vi "Old_main_broken.vi"() -> ()   [LabVIEW 2019]
uses:
  Control 3.ctl
  Control 1.ctl
  <vilib>/Analysis/3filter.llb/Filter Passband Type.ctl
  <vilib>/Analysis/5stat.llb/RMS (DBL).vi
  <vilib>/Analysis/3filter.llb/Butterworth Filter (DBL).vi
  <vilib>/Analysis/NI_AALPro.lvlib
  <vilib>/Analysis/NI_AALBase.lvlib
panel:
  out "Prubehy RMS":cluster{"rms value":dbl, "rms value":dbl}(graph)
  in  "Citlivost vypoctu frekvence":i32=10
  in  "Citlivost vypoctu frekvence":i32=50
  out "Perioda ze spektra.":dbl
  out "Perioda ze spektra":dbl
  out "Ursm":dbl format="%0.2f"
  out "Perioda z pruchodu nulou":dbl
  out "Frekvence z pruchodu nulou":dbl
  out "Urms":dbl format="%0.2f"
  out "Perioda z pruchodu nulou.":dbl
  out "Frekvence z pruchodu nulou.":dbl
  out "Frekvence ze spektra":i32
  out "Frekvence ze spektra.":i32
  out "Spektrum puvodniho signalu":cluster{dbl[], dbl[]}(graph)
  out "Spektrum prevzorkovaneho signalu":cluster{dbl[], dbl[]}(graph)
  out "Prevzorkovany signal":waveform(dbl)(graph)
  in  "Napetovy treshold":dbl=10.0
  in  "Úroven filtrace":i32
  out "Triggered signal":cluster{dbl[], "Vstupní pole":dbl[]}(graph)
  out "SamInWin":i32
  in  "Sirka okna (ms)":i32(listbox)=1
  in  "Offset":dbl format="%0.2p"
  in  "Amplituda sumu":T1
  in  "Amplituda":dbl=1.0 format="%0.2p"
  in  "Frekvence":dbl=10.0 format="%0.2p"
  out "Signal z generatoru":waveform(dbl)(graph)
  out "dt":dbl
  in  "stop":bool
  # "Parametry generatoru signalu"
  # "Hide!"
  # "Parametry navzorkovaneho signalu"
  # "Parametry prevzorkovaneho signalu"
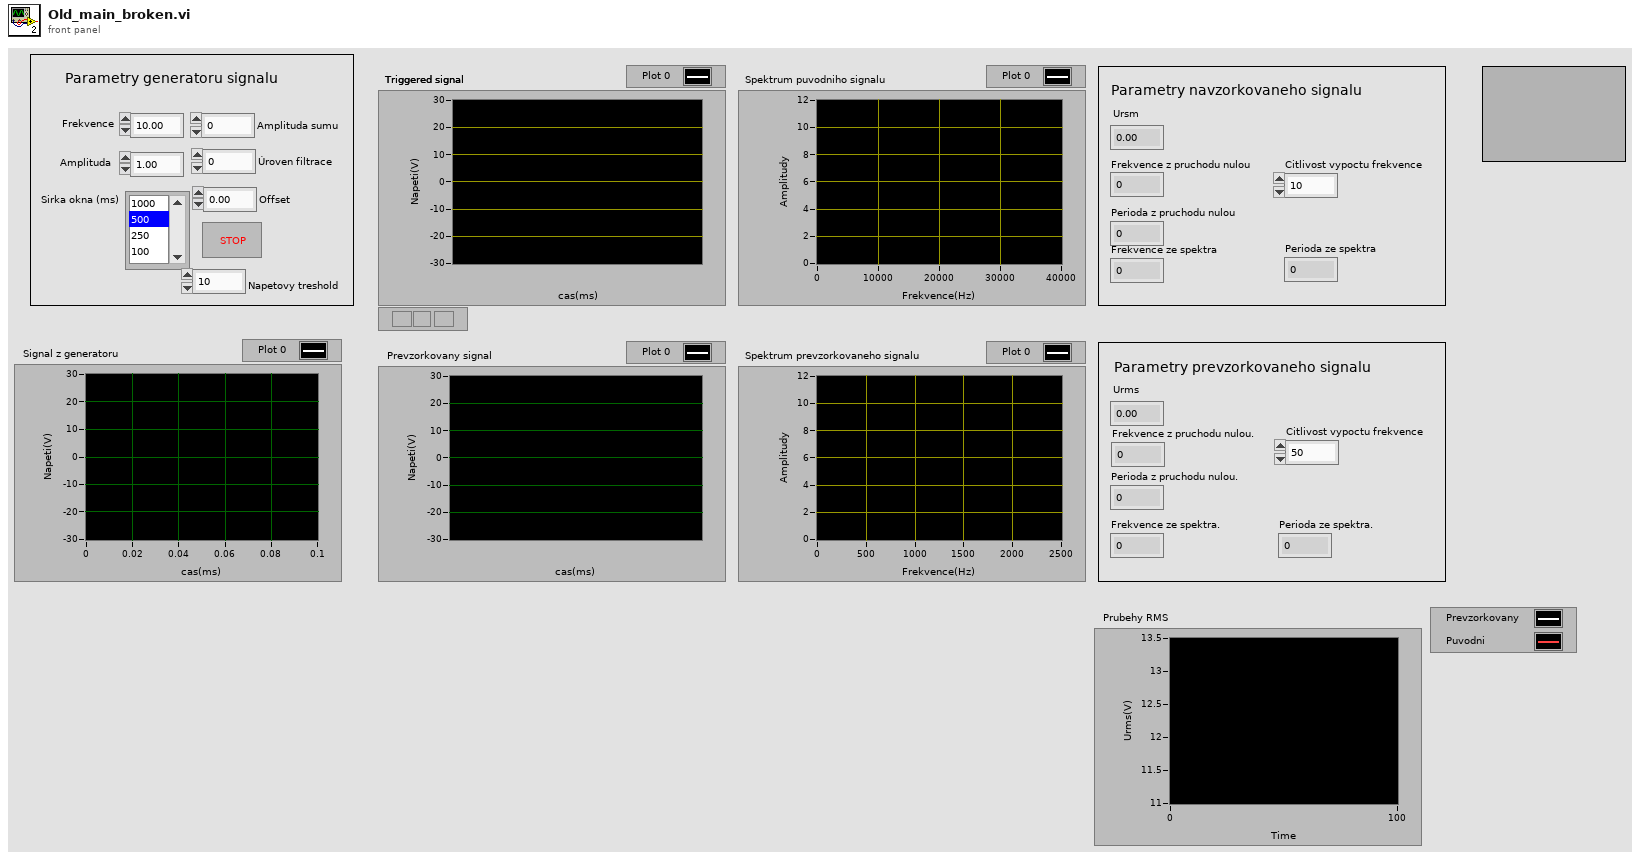
[diagram p1: front panel]
types:
  T1 = typedef "Control 3.ctl" = dbl
  T2 = enum16{"open", "open or create", "create or replace", "create", "open (read-only)"}
  T3 = cluster{"Waveform":waveform(dbl), "Waveform":waveform(dbl), "Waveform":waveform(dbl), "seconds since 1Jan1904":timestamp, bool, bool}
  T4 = typedef "Control 1.ctl" = dbl
  T5 = cluster{"name (unnamed)":string, "Variant":variant}
  T6 = typedef "NI_AALBase.lvlib/Filter Passband Type.ctl" = enum32{"Lowpass", "Highpass", "Bandpass", "Bandstop"}
  T7 = cluster{waveform(dbl), waveform(dbl), waveform(dbl), "seconds since 1Jan1904":timestamp, bool, bool}
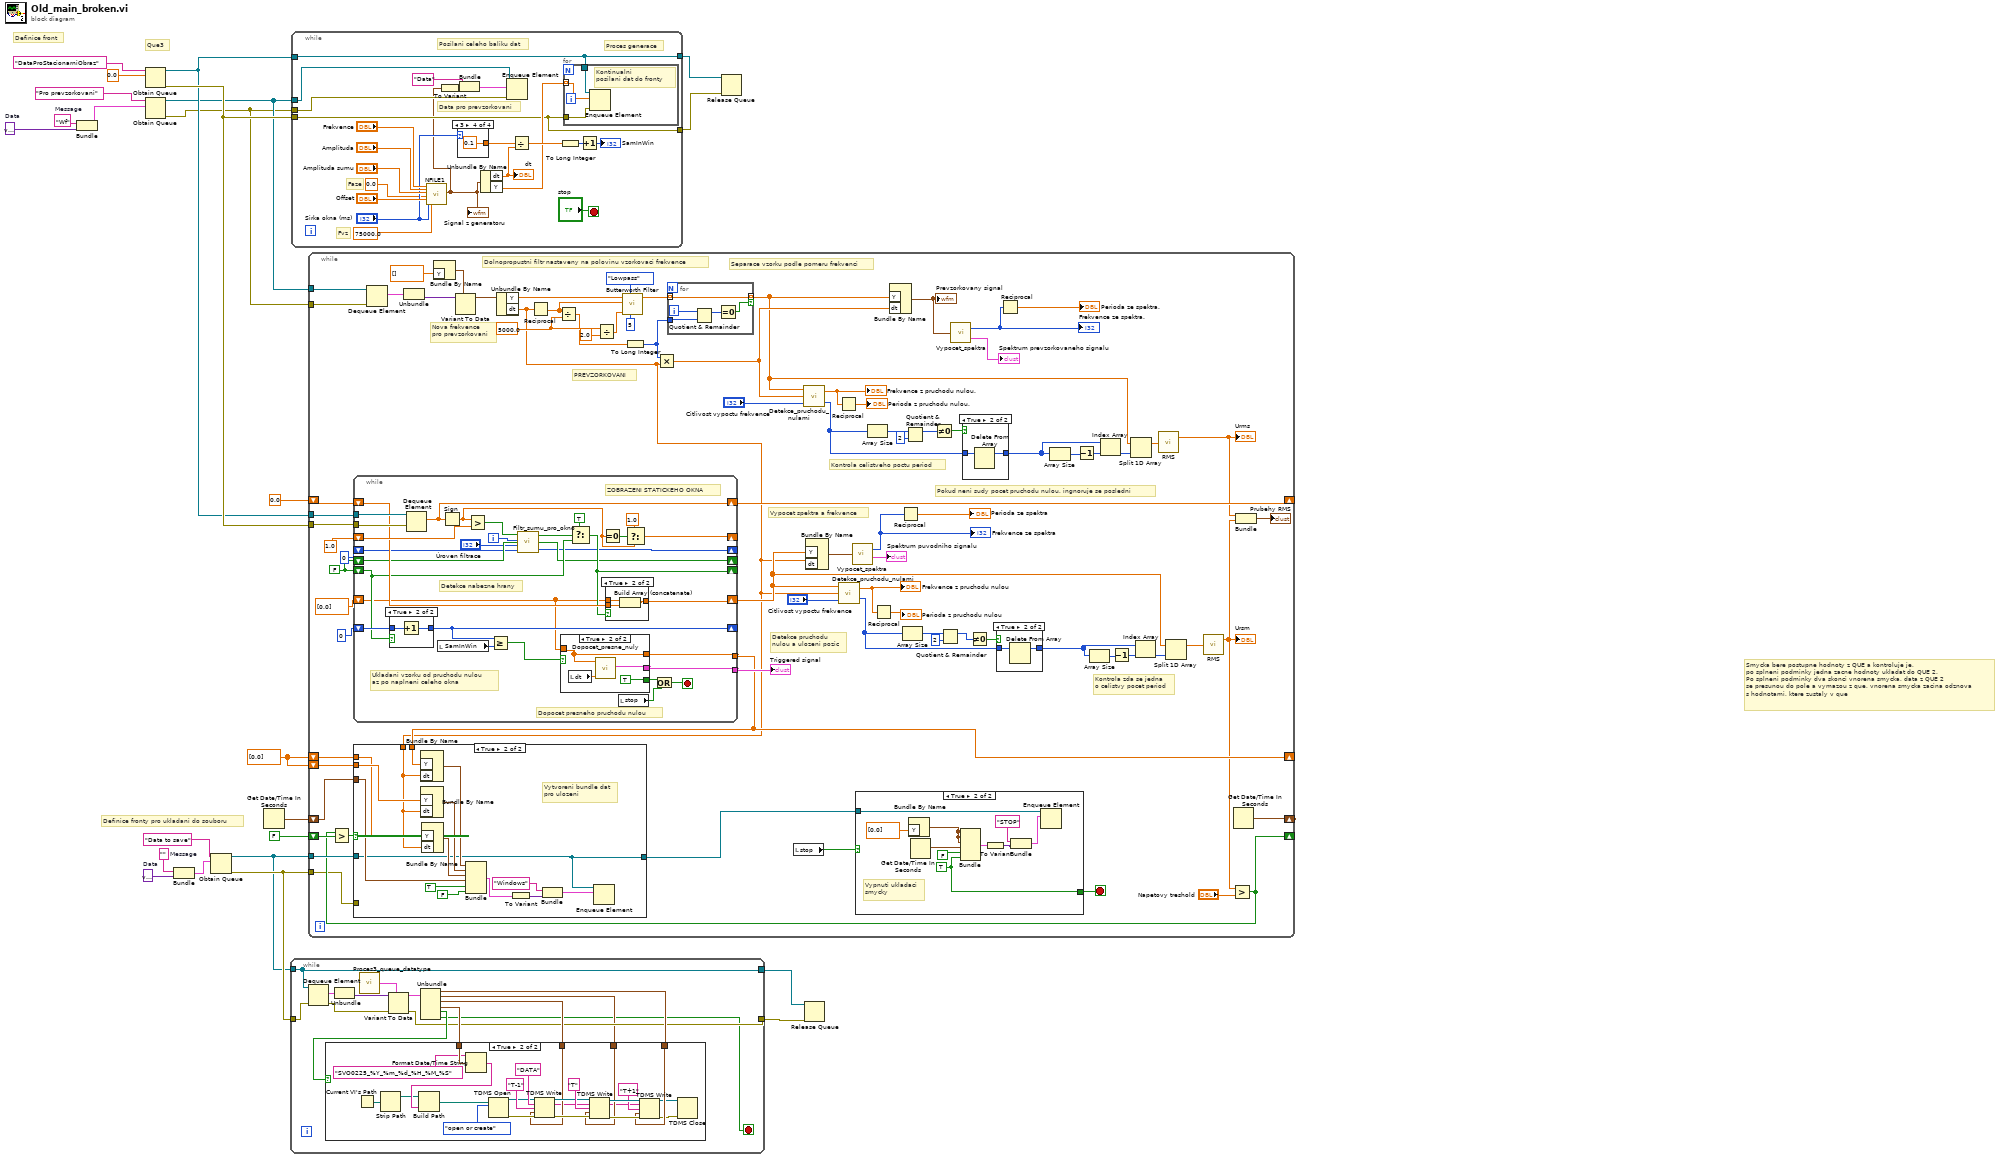
[diagram p0: block diagram]
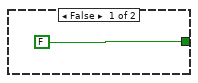
[diagram p3: hidden frame]
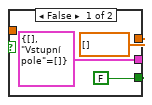
[diagram p6: hidden frame]
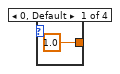
[diagram p10: hidden frame]
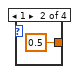
[diagram p11: hidden frame]
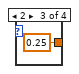
[diagram p12: hidden frame]
diagram:
  w2 = dbl[] [0.0]
  w1 = variant  # Data
  w6 = "Wf"  # Message
  w17 = variant  # Data
  w18 = ""  # Message
  # "Definice fronty pro ukladani do souboru"
  # "Definice front"
  # "Que3"
  # "Smycka bere postupne hodnoty z QUE a kontroluje je,\npo splneni podminky jedna zacne hodnoty ukladat do QUE 2.\nPo splneni podminky dva skonci vnorena smycka, data z QUE 2 \nse presunou do pole a vymazou z que, vnorena smycka zacina odznova\ns hodnotami, ktere zustaly v que"
  n1 = Bundle("Message"=w6, "Data"=w1) -> (w5:cluster{"Message":string, "Data":variant})  [unwired: 1 in]
  n2 = Obtain Queue(name (unnamed)="DataProStacionarniObraz", element data type=0.0) -> (queue out=w21:refnum<queue>, error out=w22:errorcluster)  [unwired: 3 in, 1 out]
  n3 = Obtain Queue(name (unnamed)="Pro prevzorkovani", element data type=w5) -> (queue out=w8:refnum<queue>, error out=w7:errorcluster)  [unwired: 3 in, 1 out]
  n4 = Bundle("Message"=w18, "Data"=w17) -> (w16:cluster{"Message":string, "Data":variant})  [unwired: 1 in]
  n5 = Obtain Queue(name (unnamed)="Data to save", element data type=w16) -> (queue out=w13:refnum<queue>, error out=w14:errorcluster)  [unwired: 3 in, 1 out]
  n6 = Get Date/Time In Seconds() -> (seconds since 1Jan1904=w3:timestamp)
  n7 = while {
    tunnel: w14 -> [w29]
    tunnel: w13 -> [w34]
    tunnel: [w34] -> w12
    tunnel: [w27] -> w11
    stop <- w25 stop-if-true
    n8 = Dequeue Element(queue=w34, error in (no error)=w29) -> (element=w38:cluster{"Message":string, "Data":variant}, error out=w28:errorcluster)  [unwired: 1 in, 2 out]
    n9 = Unbundle(w38) -> ("Data"=w37:variant)  [unwired: 1 out]
    n10 = call "Proces3_queue_datatype.vi"() -> ("output cluster"=w36:T3)  [unwired: 1 in]
    n11 = Variant To Data(error in=w28, type=w36, Variant=w37) -> (data=w35:T3, error out=w27:errorcluster)
    n12 = Unbundle(w35) -> ("Waveform"=w33:waveform(dbl), "Waveform"=w26:waveform(dbl), "Waveform"=w30:waveform(dbl), "seconds since 1Jan1904"=w32:timestamp, w31:bool, w25:bool)
    n13 = case shown="True" w31 {
      tunnel: w33 -> [_ w51]
      tunnel: w32 -> [_ w50]
      tunnel: w30 -> [_ w44]
      tunnel: w26 -> [_ w43]
      frame False {
      }
      frame True {
        n14 = Current VI's Path() -> (path=w62:path)
        n15 = Strip Path(path=w62) -> (stripped path=w39:path)  [unwired: 1 out]
        n16 = Format Date/Time String(time format string (%c)="SVO0225_%Y_%m_%d_%H_%M_%S", seconds (now)=w50) -> (date/time string=w61:string)  [unwired: 1 in]
        n17 = Build Path(base path=w39, name or relative path=w61) -> (appended path=w60:path)
        n18 = TDMS Open(10:T2."open or create" ("operation (0:open)"), 11:w60) -> (0:w55:errorcluster, 3:w56:refnum<k34>)  [unwired: 5 in]
        n19 = TDMS Write(0:w56, 5:"DATA" ("group name in (Untitled)"), 7:"T-1", 9:w44, 11:w55) -> (4:w45:refnum<k34>, 6:w42:string, 15:w54:errorcluster)  [unwired: 1 in, 1 out]
        n20 = TDMS Write(0:w45, 5:w42, 7:"T", 9:w43, 11:w54) -> (4:w46:refnum<k34>, 6:w40:string, 15:w52:errorcluster)  [unwired: 1 in, 1 out]
        n21 = TDMS Write(0:w46, 5:w40, 7:"T+1", 9:w51, 11:w52) -> (4:w48:refnum<k34>, 15:w49:errorcluster)  [unwired: 1 in, 2 out]
        n22 = TDMS Close(8:w49, 11:w48) -> ()  [unwired: 2 out]
      }
    }
  }
  n23 = while {
    tunnel: w22 -> [w70]
    tunnel: w21 -> [w71]
    tunnel: [w71] -> w10
    tunnel: [w70] -> w9
    tunnel: w8 -> [w69]
    tunnel: w7 -> [w68]
    stop <- "stop" stop-if-true
    # "Posilani celeho baliku dat"
    # "Data pro prevzorkovani"
    # "Proces generace"
    # "Fvz"
    # "Faze"
    n24 = call "NFILE1.vi"("Frekvence"="Frekvence", "Amplituda"="Amplituda", "Amplituda sumu"="Amplituda sumu", "Fáze"=0.0, "Offset"="Offset", "Sirka okna (ms)"="Sirka okna (ms)", "Fvz"=T4 75000.0) -> ("Waveform Graph"=w65:waveform(dbl))  [unwired: 12 in]
    "Signal z generatoru" <- w65
    n25 = To Variant(anything=w65) -> (Variant=w66:variant)
    n26 = case shown="3" "Sirka okna (ms)" {
      tunnel: [1.0 ("X Scale.Range:Maximum") 0.5 ("X Scale.Range:Maximum") 0.25 ("X Scale.Range:Maximum") 0.1 ("X Scale.Range:Maximum")] -> w77
      frame 0, Default {
      }
      frame 1 {
      }
      frame 2 {
      }
      frame 3 {
      }
    }
    n27 = Bundle("name (unnamed)"="Data", "Variant"=w66) -> (w67:T5)  [unwired: 1 in]
    n28 = Unbundle By Name(w65) -> ("dt"=w63:dbl, "Y"=w74:dbl[])
    "dt" <- w63
    n29 = Enqueue Element(queue=w69, element=w67, error in (no error)=w68) -> ()  [unwired: 1 in, 3 out]
    n30 = Divide(x=w77, y=w63) -> (x/y=w76:dbl)
    n31 = To Long Integer(number=w76) -> (32bit integer=w73:i32)
    n32 = for {
      tunnel: w70 -> [w87]
      tunnel: w71 -> [w86]
      tunnel: w74 -> [w85] mode=indexing
      # "Kontinualni\nposilani dat do fronty"
      n33 = Enqueue Element(queue=w86, element=w85, error in (no error)=w87) -> ()  [unwired: 1 in, 3 out]
    }
    n34 = Increment(x=w73) -> (x+1=→"SamInWin":i32)
  }
  n35 = while {
    tunnel: w22 -> [w173]
    tunnel: w21 -> [w172]
    shift-right: [w169] -> _
    shift-left: 0.0 -> [w168]
    shift-right: [w109] -> _
    shift-left: w2 -> [w164]
    shift-left: w2 -> [w163]
    shift-right: [w123] -> _
    shift-left: FALSE -> [w161]
    tunnel: w13 -> [w165]
    tunnel: w14 -> [w95]
    tunnel: w8 -> [w160]
    tunnel: w7 -> [w159]
    shift-right: [w100] -> _
    shift-left: w3 -> [w99]
    stop <- w94 stop-if-true
    w150 = T4 5000.0 ("Fvz")
    w97 = FALSE
    # "PREVZORKOVANI"
    # "Vypocet spektra a frekvence"
    # "Detekce pruchodu\nnulou a ulozeni pozic"
    # "Pokud neni sudy pocet pruchodu nulou, ingnoruje se posledni"
    # "Kontrola celistveho poctu period"
    # "Separace vzorku podle pomeru frekvenci"
    # "Dolnopropustni filtr nastaveny na polovinu vzorkovaci frekvence"
    # "Nova frekvence\npro prevzorkovani"
    # "Kontrola zda se jedna\no celistvy pocet period"
    n36 = while {
      tunnel: w172 -> [w234]
      tunnel: w173 -> [w233]
      shift-right: [w215] -> _
      shift-left: 1.0 -> [w232]
      shift-right: [w228] -> _
      shift-left: 0 -> [w230]
      shift-right: [w214] -> w108
      shift-left: dbl[] [0.0] -> [w211]
      tunnel: [w227] -> w170
      shift-right: [w224] -> _
      shift-left: w97 -> [w225]
      shift-right: [w213] -> w169
      shift-left: w168 -> [w226]
      shift-right: [w220] -> _
      shift-left: w97 -> [w221]
      tunnel: [w212] -> w109
      shift-right: [w209] -> _
      shift-left: 0 -> [w210]
      i -> [w222]
      stop <- w207 stop-if-true
      # "ZOBRAZENI STATICKEHO OKNA"
      # "Dopocet presneho pruchodu nulou"
      # "Detekce nabezne hrany"
      # "Ukladani vzorku od pruchodu nulou\naz po naplneni celeho okna"
      n37 = case shown="True" w225 {
        tunnel: w230 -> [w242 w244]
        tunnel: [w242 w243] -> w228
        frame False {
        }
        frame True {
          n38 = Increment(x=w244) -> (x+1=w243:i32)
        }
      }
      n39 = Dequeue Element(queue=w234, error in (no error)=w233) -> (element=w213:dbl)  [unwired: 1 in, 3 out]
      n40 = local read "SamInWin"() -> (w229:i32)
      n41 = Sign(1:w213) -> (0:w204:dbl)
      n42 = Greater?(x=w204, y=w232) -> (0:w223:bool)
      n43 = Greater Or Equal?(x=w228, y=w229) -> (x >= y?=w218:bool)
      n44 = call "Filtr_sumu_pro_okno.vi"("trig_in"=w223, "i"=w222, "Citlivost 2"="Úroven filtrace", "BShitftIn"=w210, "ShiftIn"=w221) -> ("trig_out"=w219:bool, "ShiftOut"=w220:bool, "BShiftOut"=w209:i32)
      n45 = case shown="True" w218 {
        tunnel: [FALSE TRUE] -> w206
        tunnel: w211 -> [_ w238]
        tunnel: [cluster{dbl[], "Vstupní pole":dbl[]} {[], "Vstupní pole"=[]} ("XY Graph 2") w239] -> w227
        tunnel: [dbl[] [] w238] -> w212
        frame False {
        }
        frame True {
          n46 = local read "dt"() -> (w240:dbl)
          n47 = call "Dopocet_presne_nuly.vi"("dt"=w240, "Vstupní pole"=w238) -> ("XY Graph"=w239:cluster{dbl[], "Vstupní pole":dbl[]})  [unwired: 9 in]
        }
      }
      n48 = Select(t=TRUE, s=w219, f=w225) -> (s? t:f=w224:bool)
      n49 = Equal To 0?(x=w204) -> (x = 0?=w217:bool)
      n50 = case shown="True" w224 {
        tunnel: w211 -> [w245 w248]
        tunnel: w226 -> [_ w247]
        tunnel: [w245 w246] -> w214
        frame False {
        }
        frame True {
          n51 = Build Array (concatenate)(w248, w247) -> (w246:dbl[])
        }
      }
      n52 = local read "stop"() -> (w205:bool)
      n53 = Select(t=1.0, s=w217, f=w204) -> (s? t:f=w215:dbl)
      n54 = Or(x=w206, y=w205) -> (x .or. y?=w207:bool)
    }
    "Triggered signal" <- w170
    n55 = Dequeue Element(queue=w160, error in (no error)=w159) -> (element=w158:cluster{"Message":string, "Data":variant})  [unwired: 1 in, 3 out]
    n56 = Unbundle(w158) -> ("Data"=w157:variant)  [unwired: 1 out]
    n57 = Bundle By Name("Y"=dbl[] []) -> (w156:waveform(dbl))  [unwired: 1 in]
    n58 = Variant To Data(type=w156, Variant=w157) -> (data=w155:waveform(dbl))  [unwired: 1 in, 1 out]
    n59 = Unbundle By Name(w155) -> ("Y"=w144:dbl[], "dt"=w98:dbl)
    n60 = Reciprocal(x=w98) -> (1/x=w149:dbl)
    n61 = Divide(x=w149, y=w150) -> (x/y=w147:T4)
    n62 = Divide(x=w150, y=2.0) -> (x/y=w153:T4)
    n63 = call-poly <vilib>:"Butterworth Filter.vi"("order"=5, "filter type"=Filter_Passband_Type."Lowpass", "low cutoff freq: fl"=w153, "sampling freq: fs"=w149, "X"=w144) -> ("Filtered X"=w148:dbl[])  [unwired: 3 in, 1 out]
    n64 = To Long Integer(number=w147) -> (32bit integer=w146:i32)
    n65 = Multiply(x=w146, y=w98) -> (x*y=w138:dbl)
    n66 = for {
      tunnel: w148 -> [w253] mode=indexing
      tunnel: w146 -> [w255]
      tunnel: [w253] -> w125 mode=indexing if=w252
      i -> [w256]
      n67 = Quotient & Remainder(x=w256, y=w255) -> (x-y*floor(x/y)=w254:i32)  [unwired: 1 out]
      n68 = Equal To 0?(x=w254) -> (x = 0?=w252:bool)
    }
    n69 = local read "stop"() -> (w93:bool)
    n70 = call "Detekce_pruchodu_nulami.vi"("Citlivost vypoctu frekvence"="Citlivost vypoctu frekvence", "dt 2"=w138, "array"=w125) -> ("Pole indexu pruchodu nulou"=w130:i32[], "Numeric"=w135:dbl)
    "Frekvence z pruchodu nulou." <- w135
    n71 = Bundle By Name("Y"=w108, "dt"=w98) -> (w142:waveform(dbl))  [unwired: 1 in]
    n72 = Reciprocal(x=w135) -> (1/x=→"Perioda z pruchodu nulou.":dbl)
    n73 = call "Detekce_pruchodu_nulami.vi"("Citlivost vypoctu frekvence"="Citlivost vypoctu frekvence", "dt 2"=w98, "array"=w108) -> ("Pole indexu pruchodu nulou"=w115:i32[], "Numeric"=w120:dbl)
    "Frekvence z pruchodu nulou" <- w120
    n74 = call "Vypocet_spektra.vi"("waveform"=w142) -> ("Frekvence"=w107:i32, "XY Graph"=→"Spektrum puvodniho signalu":cluster{dbl[], dbl[]})
    "Frekvence ze spektra" <- w107
    n75 = Array Size(array=w130) -> (size(s)=w133:i32)
    n76 = Reciprocal(x=w120) -> (1/x=→"Perioda z pruchodu nulou":dbl)
    n77 = Bundle By Name("Y"=w125, "dt"=w138) -> (w143:waveform(dbl))  [unwired: 1 in]
    "Prevzorkovany signal" <- w143
    n78 = Reciprocal(x=w107) -> (1/x=→"Perioda ze spektra":dbl)
    n79 = Array Size(array=w115) -> (size(s)=w118:i32)
    n80 = Quotient & Remainder(x=w133, y=2) -> (x-y*floor(x/y)=w134:i32)  [unwired: 1 out]
    n81 = Not Equal To 0?(x=w134) -> (x != 0?=w131:bool)
    n82 = Quotient & Remainder(x=w118, y=2) -> (x-y*floor(x/y)=w119:i32)  [unwired: 1 out]
    n83 = call "Vypocet_spektra.vi"("waveform"=w143) -> ("Frekvence"=w104:i32, "XY Graph"=→"Spektrum prevzorkovaneho signalu":cluster{dbl[], dbl[]})
    "Frekvence ze spektra." <- w104
    n84 = case shown="True" w131 {
      tunnel: w130 -> [w249 w251]
      tunnel: [w249 w250] -> w127
      frame False {
      }
      frame True {
        n85 = Delete From Array(array=w251) -> (array with subset deleted=w250:i32[])  [unwired: 2 in, 1 out]
      }
    }
    n86 = Not Equal To 0?(x=w119) -> (x != 0?=w116:bool)
    n87 = case shown="True" w116 {
      tunnel: w115 -> [w185 w187]
      tunnel: [w185 w186] -> w112
      frame False {
      }
      frame True {
        n88 = Delete From Array(array=w187) -> (array with subset deleted=w186:i32[])  [unwired: 2 in, 1 out]
      }
    }
    n89 = Reciprocal(x=w104) -> (1/x=→"Perioda ze spektra.":dbl)
    n90 = Array Size(array=w127) -> (size(s)=w129:i32)
    n91 = Decrement(x=w129) -> (x-1=w128:i32)
    n92 = Array Size(array=w112) -> (size(s)=w114:i32)
    n93 = Index Array(array=w127, index=w128) -> (element=w126:i32)
    n94 = Decrement(x=w114) -> (x-1=w113:i32)
    n95 = Split 1D Array(array=w125, index=w126) -> (first subarray=w124:dbl[])  [unwired: 1 out]
    n96 = Index Array(array=w112, index=w113) -> (element=w111:i32)
    n97 = call-poly <vilib>:"RMS.vi"("X"=w124) -> ("rms value"=w102:dbl)  [unwired: 1 out]
    "Urms" <- w102
    n98 = Split 1D Array(array=w108, index=w111) -> (first subarray=w110:dbl[])  [unwired: 1 out]
    n99 = call-poly <vilib>:"RMS.vi"("X"=w110) -> ("rms value"=w103:dbl)  [unwired: 1 out]
    "Ursm" <- w103
    n100 = Greater?(x=w103, y="Napetovy treshold") -> (0:w123:bool)
    n101 = Greater?(x=w123, y=w161) -> (0:w162:bool)
    n102 = case shown="True" w162 {
      tunnel: w165 -> [w188 w189]
      tunnel: w164 -> [_ w196]
      tunnel: w163 -> [_ w197]
      tunnel: w109 -> [_ w198]
      tunnel: w99 -> [_ w199]
      tunnel: w98 -> [_ w195]
      tunnel: w95 -> [_ _]
      tunnel: [w188 w189] -> w92
      frame False {
      }
      frame True {
        # "Vytvoreni bundle dat\npro ulozeni"
        n103 = Bundle By Name("Y"=w198, "dt"=w195) -> (w192:waveform(dbl))  [unwired: 1 in]
        n104 = Bundle By Name("Y"=w197, "dt"=w195) -> (w193:waveform(dbl))  [unwired: 1 in]
        n105 = Bundle By Name("Y"=w196, "dt"=w195) -> (w194:waveform(dbl))  [unwired: 1 in]
        n106 = Bundle(w192, w193, w194, "seconds since 1Jan1904"=w199, TRUE, FALSE) -> (w201:T7)  [unwired: 1 in]
        n107 = To Variant(anything=w201) -> (Variant=w202:variant)
        n108 = Bundle("Windows", "Variant"=w202) -> (w200:cluster{string, "Variant":variant})  [unwired: 1 in]
        n109 = Enqueue Element(queue=w189, element=w200) -> ()  [unwired: 2 in, 3 out]
      }
    }
    n110 = case shown="True" w93 {
      tunnel: [FALSE w181] -> w94
      tunnel: w92 -> [_ w179]
      frame False {
      }
      frame True {
        w181 = TRUE
        # "Vypnuti ukladaci\nsmycky"
        n111 = Bundle By Name("Y"=dbl[] [0.0]) -> (w184:waveform(dbl))  [unwired: 1 in]
        n112 = Get Date/Time In Seconds() -> (seconds since 1Jan1904=w183:timestamp)
        n113 = Bundle(w184, w184, w184, "seconds since 1Jan1904"=w183, FALSE, w181) -> (w177:T7)  [unwired: 1 in]
        n114 = To Variant(anything=w177) -> (Variant=w178:variant)
        n115 = Bundle("STOP", "Variant"=w178) -> (w175:cluster{string, "Variant":variant})  [unwired: 1 in]
        n116 = Enqueue Element(queue=w179, element=w175) -> ()  [unwired: 2 in, 3 out]
      }
    }
    n117 = Get Date/Time In Seconds() -> (seconds since 1Jan1904=w100:timestamp)
    n118 = Bundle("rms value"=w102, "rms value"=w103) -> (→"Prubehy RMS":cluster{"rms value":dbl, "rms value":dbl})  [unwired: 1 in]
  }
  n119 = Release Queue(queue=w10, error in (no error)=w9) -> ()  [unwired: 1 in, 3 out]
  n120 = Release Queue(queue=w12, error in (no error)=w11) -> ()  [unwired: 1 in, 3 out]
